vi "goInCircles.vi"(8 "error in (no error)":errorcluster, 11 "StationKeeping in":refnum<class "StationKeeping.lvclass">) -> (0 "error out":errorcluster, 2 "No Sail Circles":T1[](array[typedef]), 3 "StationKeeping out":refnum<class "StationKeeping.lvclass">)   [LabVIEW 2011, in "StationKeeping.lvclass"]
doc: "makes 8 No Sail Zones. One one each corner of the station, and one on the midpoint of each edge. The circle sizes are 1/3 of the edge length of the station (1/4 would make them just barely close the station). This keeps the boat from being able to leave the station, although it is not very consistent in how close it allows the boat to come to the edge.\n\nNote: this VI is named stupidly. I don't know what I was thinking."
uses:
  StationKeeping.lvclass
  2 Typedefs/UTM Circle.ctl
  StationKeeping.lvclass/StationKeeping.ctl
panel:
  in  "Radius of No Sail Zones":dbl=3.0
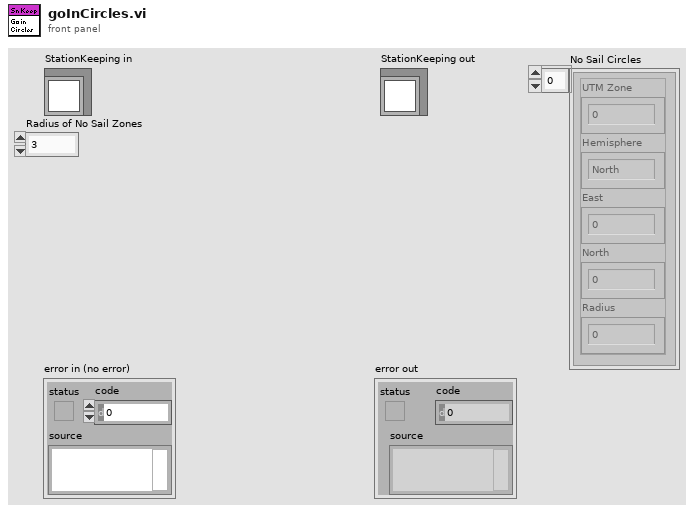
[diagram p1: front panel]
types:
  T1 = typedef "UTM Circle.ctl" = cluster{"UTM Zone":dbl, "Hemisphere":enum16{"North", "South"}, "East":dbl, "North":dbl, "Radius":dbl}
  T2 = typedef "UTM Location.ctl" = cluster{"UTM Zone":dbl, "Hemisphere":enum16{"North", "South"}, "East":dbl, "North":dbl}
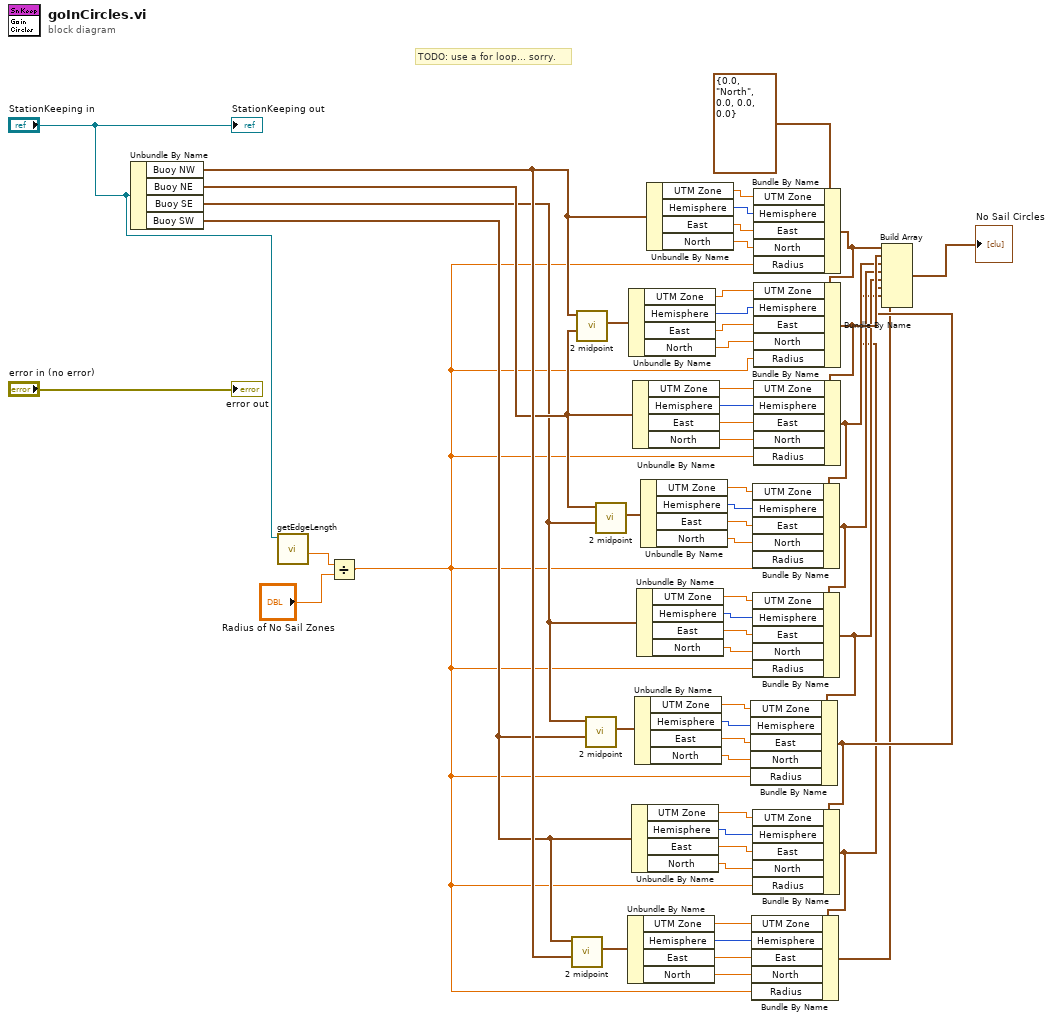
[diagram p0: block diagram]
diagram:
  # "TODO: use a for loop... sorry."
  n1 = Unbundle By Name("StationKeeping in") -> ("Buoy NW"=w8:T2, "Buoy NE"=w7:T2, "Buoy SE"=w6:T2, "Buoy SW"=w5:T2)
  n2 = call "getEdgeLength.vi"("StationKeeping in"="StationKeeping in") -> ("Edge Length"=w2:dbl)  [unwired: 9 in, 1 out]
  n3 = Divide(x=w2, y="Radius of No Sail Zones") -> (x/y=w3:dbl)
  n4 = call "2 midpoint.vi"("UTM 2"=w8, "UTM 1"=w5) -> ("Midpoint"=w12:T2)  [unwired: 8 in, 1 out]
  n5 = call "2 midpoint.vi"("UTM 2"=w7, "UTM 1"=w8) -> ("Midpoint"=w9:T2)  [unwired: 8 in, 1 out]
  n6 = call "2 midpoint.vi"("UTM 2"=w5, "UTM 1"=w6) -> ("Midpoint"=w11:T2)  [unwired: 8 in, 1 out]
  n7 = call "2 midpoint.vi"("UTM 2"=w6, "UTM 1"=w7) -> ("Midpoint"=w10:T2)  [unwired: 8 in, 1 out]
  n8 = Unbundle By Name(w12) -> ("UTM Zone"=w33:dbl, "Hemisphere"=w34:enum16{"North", "South"}, "East"=w35:dbl, "North"=w36:dbl)
  n9 = Unbundle By Name(w9) -> ("UTM Zone"=w40:dbl, "Hemisphere"=w39:enum16{"North", "South"}, "East"=w38:dbl, "North"=w37:dbl)
  n10 = Unbundle By Name(w5) -> ("UTM Zone"=w29:dbl, "Hemisphere"=w30:enum16{"North", "South"}, "East"=w31:dbl, "North"=w32:dbl)
  n11 = Unbundle By Name(w7) -> ("UTM Zone"=w13:dbl, "Hemisphere"=w14:enum16{"North", "South"}, "East"=w15:dbl, "North"=w16:dbl)
  n12 = Unbundle By Name(w11) -> ("UTM Zone"=w25:dbl, "Hemisphere"=w26:enum16{"North", "South"}, "East"=w27:dbl, "North"=w28:dbl)
  n13 = Unbundle By Name(w6) -> ("UTM Zone"=w21:dbl, "Hemisphere"=w22:enum16{"North", "South"}, "East"=w23:dbl, "North"=w24:dbl)
  n14 = Unbundle By Name(w10) -> ("UTM Zone"=w17:dbl, "Hemisphere"=w18:enum16{"North", "South"}, "East"=w19:dbl, "North"=w20:dbl)
  n15 = Unbundle By Name(w8) -> ("UTM Zone"=w52:dbl, "Hemisphere"=w51:enum16{"North", "South"}, "East"=w50:dbl, "North"=w49:dbl)
  n16 = Bundle By Name(cluster=T1 {"UTM Zone"=0.0, "Hemisphere"=enum."North", "East"=0.0, "North"=0.0, "Radius"=0.0} ("UTM Location"), "UTM Zone"=w52, "Hemisphere"=w51, "East"=w50, "North"=w49, "Radius"=w3) -> (w48:T1)
  n17 = Bundle By Name(cluster=w48, "UTM Zone"=w40, "Hemisphere"=w39, "East"=w38, "North"=w37, "Radius"=w3) -> (w47:T1)
  n18 = Bundle By Name(cluster=w47, "UTM Zone"=w13, "Hemisphere"=w14, "East"=w15, "North"=w16, "Radius"=w3) -> (w46:T1)
  n19 = Bundle By Name(cluster=w46, "UTM Zone"=w17, "Hemisphere"=w18, "East"=w19, "North"=w20, "Radius"=w3) -> (w45:T1)
  n20 = Bundle By Name(cluster=w45, "UTM Zone"=w21, "Hemisphere"=w22, "East"=w23, "North"=w24, "Radius"=w3) -> (w44:T1)
  n21 = Bundle By Name(cluster=w44, "UTM Zone"=w25, "Hemisphere"=w26, "East"=w27, "North"=w28, "Radius"=w3) -> (w43:T1)
  n22 = Bundle By Name(cluster=w43, "UTM Zone"=w29, "Hemisphere"=w30, "East"=w31, "North"=w32, "Radius"=w3) -> (w41:T1)
  n23 = Bundle By Name(cluster=w41, "UTM Zone"=w33, "Hemisphere"=w34, "East"=w35, "North"=w36, "Radius"=w3) -> (w42:T1)
  n24 = Build Array(w48, w47, w46, w45, w44, w43, w41, w42) -> (→"No Sail Circles":T1[])
  "error out" <- "error in (no error)"
  "StationKeeping out" <- "StationKeeping in"
